vi "traceFileIO_traces_nr.vi"(0 "path":path, 5 "error in (no error)":errorcluster, 7 "dialog (empty path)":bool) -> (13 "cancelled":bool, 14 "actual path":path, 17 "traces nr":i32, 19 "error out":errorcluster)   [LabVIEW 2010, in "OSA.lvclass"]
doc: "Check nr of traces saved in file, (fileformat must be spf2)."
uses:
  OSA.lvclass
  OSA20X_misc.lvlib
  FTSLib.dll
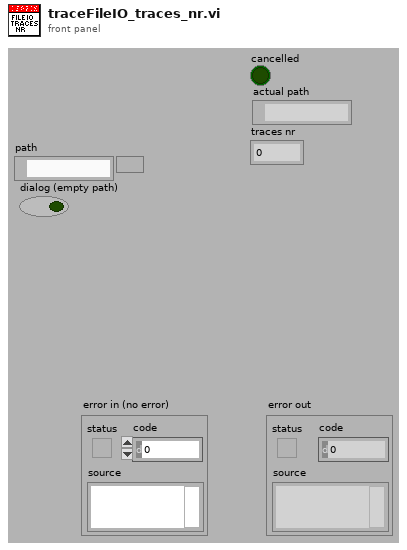
[diagram p1: front panel]
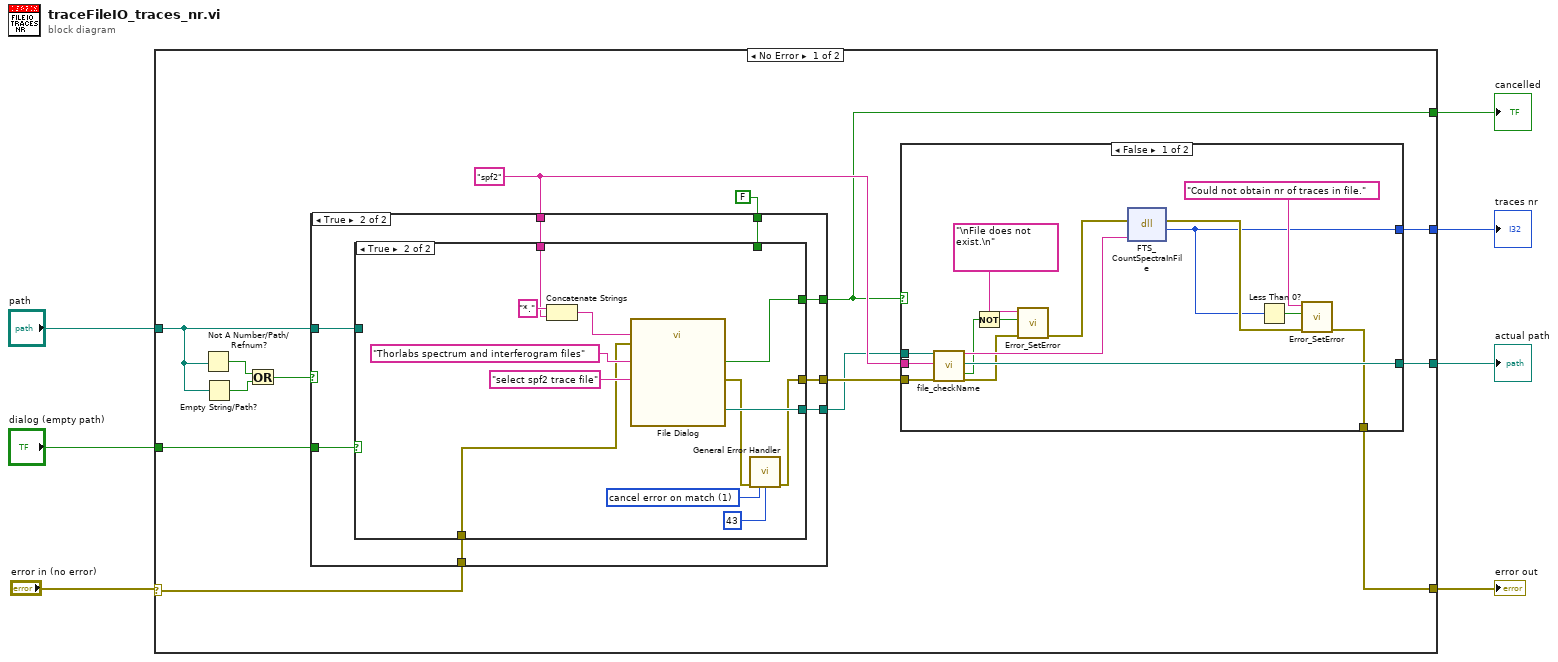
[diagram p0: block diagram]
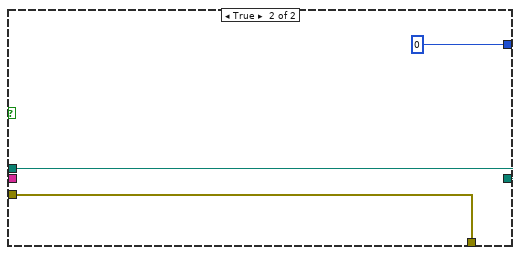
[diagram p2: hidden frame]
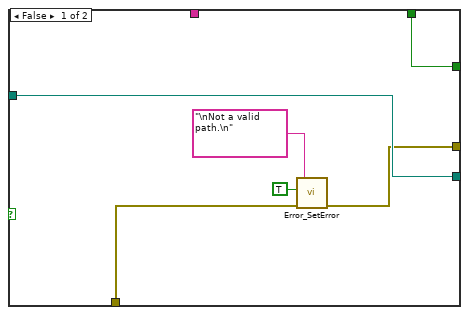
[diagram p4: hidden frame]
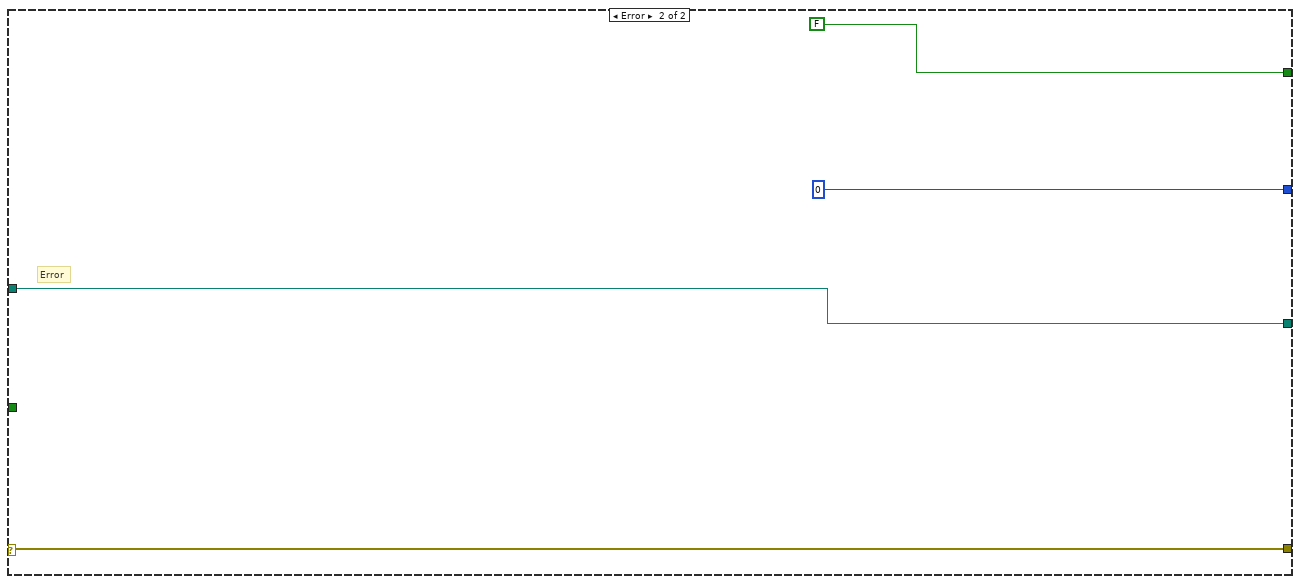
[diagram p5: hidden frame]
diagram:
  n1 = case shown="No Error" "error in (no error)" {
    selector: "error in (no error)" -> [w13 w72]
    tunnel: [w11 w72] -> w7
    tunnel: "path" -> [w18 w70]
    tunnel: "dialog (empty path)" -> [w17 _]
    tunnel: [w8 FALSE ("cancelled")] -> w3
    tunnel: [w12 w70] -> w2
    tunnel: [w10 0 ("returnVal")] -> w1
    frame No Error {
      w15 = "spf2" ("filename extension")
      n2 = Not A Number/Path/Refnum?(number/path/refnum=w18) -> (NaN/Path/Refnum?=w20:bool)
      n3 = Empty String/Path?(string/path=w18) -> (empty?=w21:bool)
      n4 = Or(x=w20, y=w21) -> (x .or. y?=w19:bool)
      n5 = case shown="True" w19 {
        tunnel: w18 -> [w42 w47]
        tunnel: w17 -> [_ w50]
        tunnel: [w40 w48] -> w8
        tunnel: [w42 w49] -> w14
        tunnel: [w41 w46] -> w16
        tunnel: w15 -> [_ w45]
        tunnel: w13 -> [w41 w44]
        tunnel: FALSE ("cancelled") -> [w40 w43]
        frame False {
        }
        frame True {
          n6 = case shown="True" w50 {
            tunnel: [w54 w66] -> w49
            tunnel: [w51 w65] -> w48
            tunnel: w47 -> [w54 _]
            tunnel: [w53 w61] -> w46
            tunnel: w45 -> [_ w58]
            tunnel: w44 -> [w52 w57]
            tunnel: w43 -> [w51 _]
            frame False {
              n7 = call "Error_SetError.vi"("error in"=w52, "status (true)"=TRUE, "source(\"\")"="\nNot a valid path.\n" ("source(\"\")")) -> ("error out"=w53:errorcluster)  [unwired: 4 in]
            }
            frame True {
              w64 = 1 items=["no exception", "cancel error on match", "set error on match"] ("[exception action] (none:0)")
              n8 = Concatenate Strings("*." ("string"), w58) -> (w60:string)
              n9 = call "File Dialog"("prompt"="select spf2 trace file", "default name"=w60, "error in"=w57, "pattern label"="Thorlabs spectrum and interferogram files") -> ("selected path"=w66:path, "cancelled"=w65:bool, "error out"=w62:errorcluster)  [unwired: 8 in, 1 out]
              n10 = call <vilib>:"General Error Handler.vi"("error in (no error)"=w62, "[exception action] (none:0)"=w64, "[exception code]"=43) -> ("error out"=w61:errorcluster)  [unwired: 8 in, 4 out]
            }
          }
        }
      }
      n11 = case shown="False" w8 {
        tunnel: w16 -> [w36 w39]
        tunnel: w15 -> [w35 _]
        tunnel: w14 -> [w33 w37]
        tunnel: [w32 w37] -> w12
        tunnel: [w30 w39] -> w11
        tunnel: [w22 0 ("returnVal")] -> w10
        frame False {
          n12 = call "file_checkName.vi"("path"=w33, "filename extension"=w35, "error in (no error)"=w36) -> ("path string out"=w34:string, "actual path"=w32:path, "exist"=w26:bool, "error out"=w28:errorcluster)  [unwired: 13 in]
          n13 = Not(x=w26) -> (.not. x?=w24:bool)
          n14 = call "Error_SetError.vi"("error in"=w28, "status (true)"=w24, "source(\"\")"="\nFile does not exist.\n" ("source(\"\")")) -> ("error out"=w27:errorcluster)  [unwired: 4 in]
          n15 = dll-call lib="FTSLib.dll" fn="FTS_CountSpectraInFile"(error in=w27, "filenameAndPath"=w34) -> (error out=w31:errorcluster, "returnVal"=w22:i32)  [unwired: 3 in, 1 out]
          n16 = Less Than 0?(x=w22) -> (x < 0?=w23:bool)
          n17 = call "Error_SetError.vi"("error in"=w31, "status (true)"=w23, "source(\"\")"="Could not obtain nr of traces in file." ("source(\"\")")) -> ("error out"=w30:errorcluster)  [unwired: 4 in]
        }
        frame True {
        }
      }
    }
    frame Error {
      # "Error"
    }
  }
  "error out" <- w7
  "cancelled" <- w3
  "actual path" <- w2
  "traces nr" <- w1
